vi "Enregistre.vi"(11 "cluster de sortie 2":T1) -> ()   [LabVIEW 2017]
uses:
  C:/Users/h16034903/Downloads/Masure_Henry_projet.llb/Variable globale 1.vi
panel:
  in  "Message":string
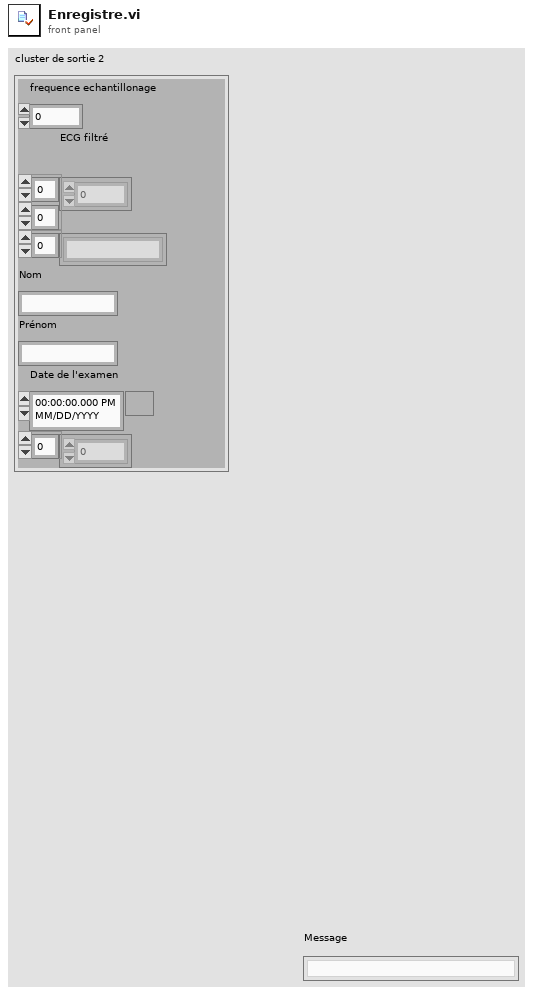
[diagram p1: front panel]
types:
  T1 = cluster{"frequence echantillonage":dbl, "ECG filtré\n":dbl[][], string[], "Nom":string, "Prénom":string, "Date de l'examen":timestamp, i32[]}
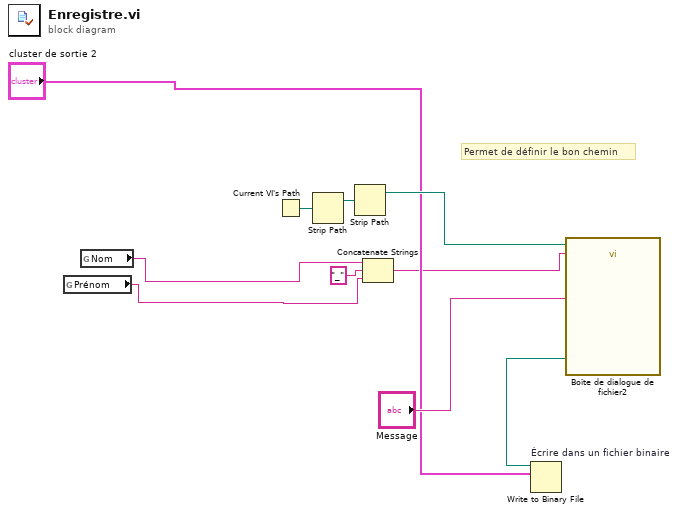
[diagram p0: block diagram]
diagram:
  # "Permet de définir le bon chemin"
  n1 = global read "Variable globale 1.vi" "Prénom"() -> (w2:string)
  n2 = global read "Variable globale 1.vi" "Nom"() -> (w3:string)
  n3 = Current VI's Path() -> (path=w9:path)
  n4 = Strip Path(path=w9) -> (stripped path=w8:path)  [unwired: 1 out]
  n5 = Strip Path(path=w8) -> (stripped path=w7:path)  [unwired: 1 out]
  n6 = Concatenate Strings(w3, "_" ("chaîne"), w2) -> (w1:string)
  n7 = call "Boîte de dialogue de fichier2"("start path"=w7, "prompt"="Message", "default name"=w1) -> ("selected path"=w10:path)  [unwired: 9 in, 3 out]
  n8 = Write to Binary File "Écrire dans un fichier binaire"(file (use dialog)=w10, data="cluster de sortie 2") -> ()  [unwired: 4 in, 3 out]
